vi "Execute Menu Item.vi"(7 "Device Ref in":T1 format="%.0x", 8 "error in (no error)":errorcluster, 9 "Coords":T2, 10 "ItemTag":string, 11 "CtlRef":refnum<vi>) -> (0 "error out":errorcluster)   [LabVIEW 2014, in "SLSC configuration System Explorer.lvlib"]
uses:
  SLSC configuration System Explorer.lvlib
  <vilib>/Utility/miscctls.llb/LVPoint32TypeDef.ctl
  <vilib>/NI Veristand/Custom Device API/Custom Device Item Ref.ctl
  Type Defs/Card Position.ctl
  Shared/SPI Utility/Slot #.ctl
  <vilib>/NI Veristand/Custom Device Tools/Custom Device Utility Library/NI VeriStand - Search for Item by Name.vi
  <vilib>/NI Veristand/Custom Device API/Custom Device API.lvlib
  <vilib>/NI Veristand/Custom Device Tools/Custom Device Utility Library/Custom Device Utility Library.lvlib
  Shared/SLSC configuration Shared.lvlib
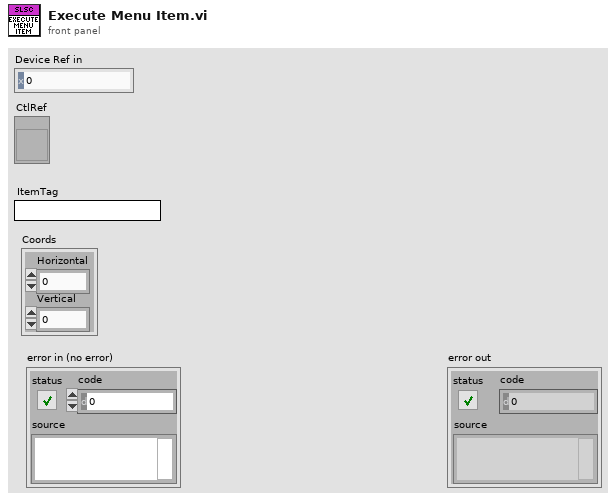
[diagram p1: front panel]
types:
  T1 = typedef "Custom Device API.lvlib/Custom Device Item Ref.ctl" = u64
  T2 = typedef "LVPoint32TypeDef.ctl" = cluster{"Horizontal":i32, "Vertical":i32}
  T3 = typedef "SLSC configuration Shared.lvlib/Card Position.ctl" = cluster{"Rack #":u8, "Slot #":T4}
  T4 = typedef "SLSC configuration Shared.lvlib/Slot #.ctl" = u8
  T5 = typedef "LVRowAndColumnTypeDef.ctl" = cluster{"Row":i32, "Column":i32}
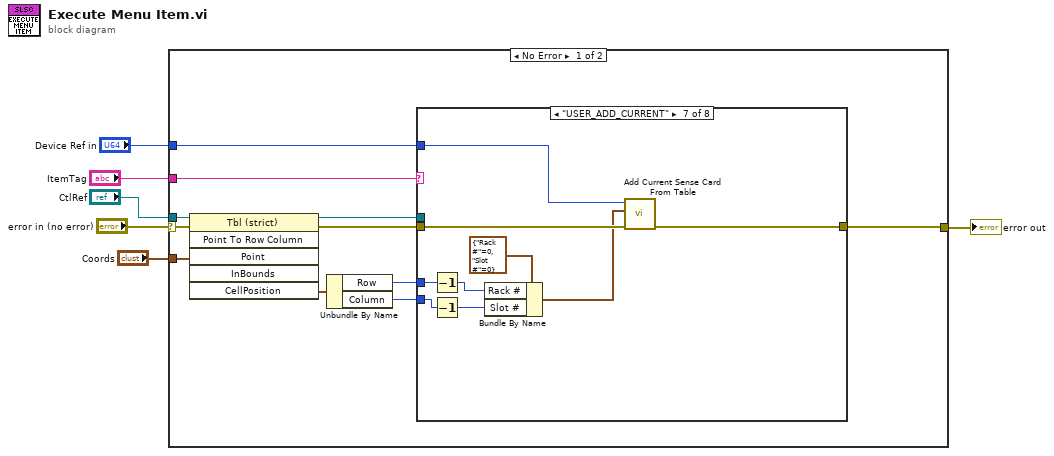
[diagram p0: block diagram]
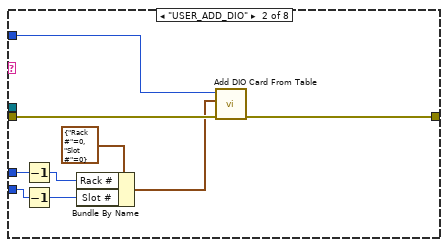
[diagram p3: hidden frame]
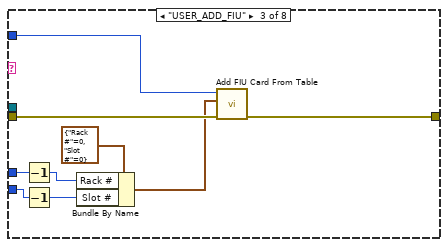
[diagram p4: hidden frame]
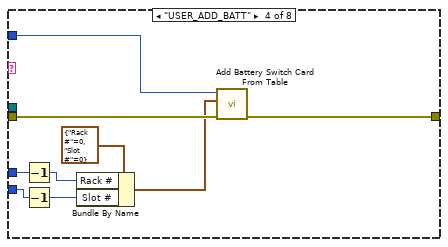
[diagram p5: hidden frame]
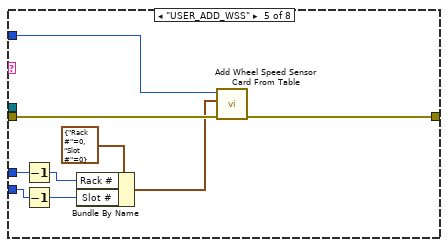
[diagram p6: hidden frame]
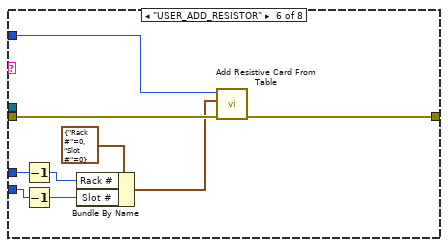
[diagram p7: hidden frame]
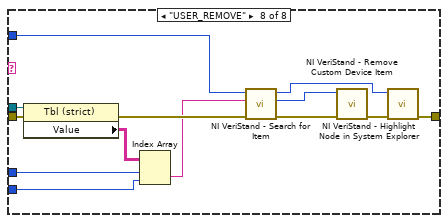
[diagram p8: hidden frame]
diagram:
  n1 = case shown="No Error" "error in (no error)" {
    selector: "error in (no error)" -> [w15 w86]
    tunnel: "ItemTag" -> [w17 _]
    tunnel: "CtlRef" -> [w16 _]
    tunnel: "Coords" -> [w14 _]
    tunnel: "Device Ref in" -> [w8 _]
    tunnel: [w7 w86] -> w1
    frame No Error {
      n2 = invoke class="Tbl (strict)" method="Point To Row Column"(reference=w16, error in=w15, "Point"=w14) -> (reference out=w13:refnum<vi>, error out=w12:errorcluster, "CellPosition"=w11:T5)  [unwired: 3 in, 3 out]
      n3 = Unbundle By Name(w11) -> ("Row"=w10:i32, "Column"=w9:i32)
      n4 = case shown="\"USER_ADD_CURRENT\"" w17 {
        tunnel: w13 -> [_ _ _ _ _ _ _ w85]
        tunnel: w12 -> [w18 w22 w31 w40 w49 w58 w67 w84]
        tunnel: w10 -> [_ w26 w35 w44 w53 w62 w71 w82]
        tunnel: w9 -> [_ w25 w34 w43 w52 w61 w70 w81]
        tunnel: w8 -> [_ w19 w29 w38 w47 w56 w65 w79]
        tunnel: [w18 w21 w30 w39 w48 w57 w66 w73] -> w7
        frame Default {
        }
        frame "USER_ADD_DIO" {
          n5 = Decrement(x=w26) -> (x-1=w24:i32)
          n6 = Decrement(x=w25) -> (x-1=w23:i32)
          n7 = Bundle By Name(cluster=T3 {"Rack #"=0, "Slot #"=0} ("Card Position"), "Rack #"=w24, "Slot #"=w23) -> (w20:T3)
          n8 = call "Add DIO Card From Table.vi"("error in (no error)"=w22, "Card Position"=w20, "Node Ptr"=w19) -> ("error out"=w21:errorcluster)  [unwired: 8 in]
        }
        frame "USER_ADD_FIU" {
          n9 = Decrement(x=w35) -> (x-1=w33:i32)
          n10 = Decrement(x=w34) -> (x-1=w32:i32)
          n11 = Bundle By Name(cluster=T3 {"Rack #"=0, "Slot #"=0} ("Card Position"), "Rack #"=w33, "Slot #"=w32) -> (w28:T3)
          n12 = call "Add FIU Card From Table.vi"("error in (no error)"=w31, "Card Position"=w28, "Node Ptr"=w29) -> ("error out"=w30:errorcluster)  [unwired: 8 in]
        }
        frame "USER_ADD_BATT" {
          n13 = Decrement(x=w44) -> (x-1=w42:i32)
          n14 = Decrement(x=w43) -> (x-1=w41:i32)
          n15 = Bundle By Name(cluster=T3 {"Rack #"=0, "Slot #"=0} ("Card Position"), "Rack #"=w42, "Slot #"=w41) -> (w37:T3)
          n16 = call "Add Battery Switch Card From Table.vi"("error in (no error)"=w40, "Card Position"=w37, "Node Ptr"=w38) -> ("error out"=w39:errorcluster)  [unwired: 8 in]
        }
        frame "USER_ADD_WSS" {
          n17 = Decrement(x=w53) -> (x-1=w51:i32)
          n18 = Decrement(x=w52) -> (x-1=w50:i32)
          n19 = Bundle By Name(cluster=T3 {"Rack #"=0, "Slot #"=0} ("Card Position"), "Rack #"=w51, "Slot #"=w50) -> (w46:T3)
          n20 = call "Add Wheel Speed Sensor Card From Table.vi"("error in (no error)"=w49, "Card Position"=w46, "Node Ptr"=w47) -> ("error out"=w48:errorcluster)  [unwired: 8 in]
        }
        frame "USER_ADD_RESISTOR" {
          n21 = Decrement(x=w62) -> (x-1=w60:i32)
          n22 = Decrement(x=w61) -> (x-1=w59:i32)
          n23 = Bundle By Name(cluster=T3 {"Rack #"=0, "Slot #"=0} ("Card Position"), "Rack #"=w60, "Slot #"=w59) -> (w55:T3)
          n24 = call "Add Resistive Card From Table.vi"("error in (no error)"=w58, "Card Position"=w55, "Node Ptr"=w56) -> ("error out"=w57:errorcluster)  [unwired: 8 in]
        }
        frame "USER_ADD_CURRENT" {
          n25 = Decrement(x=w71) -> (x-1=w69:i32)
          n26 = Decrement(x=w70) -> (x-1=w68:i32)
          n27 = Bundle By Name(cluster=T3 {"Rack #"=0, "Slot #"=0} ("Card Position"), "Rack #"=w69, "Slot #"=w68) -> (w64:T3)
          n28 = call "Add Current Sense Card From Table.vi"("error in (no error)"=w67, "Card Position"=w64, "Node Ptr"=w65) -> ("error out"=w66:errorcluster)  [unwired: 8 in]
        }
        frame "USER_REMOVE" {
          n29 = property class="Tbl (strict)"(reference=w85, error in=w84) -> (error out=w80:errorcluster, "Value"=w83:string[][])  [unwired: 1 out]
          n30 = Index Array(array=w83, index (row)=w82, index (col)=w81) -> (element=w78:string)
          n31 = call-poly <vilib>:"NI VeriStand - Search for Item.vi"("error in"=w80, "Item Name"=w78, "Section Ref in"=w79) -> ("error out"=w77:errorcluster, "Item Ref"=w76:T1, "Section Ref out"=w74:T1)  [unwired: 5 in, 1 out]
          n32 = call <vilib>:"NI VeriStand - Remove Custom Device Item.vi"("error in (no error)"=w77, "Item Ref in"=w76) -> ("error out"=w75:errorcluster)  [unwired: 8 in, 1 out]
          n33 = call <vilib>:"NI VeriStand - Highlight Node in System Explorer.vi"("error in (no error)"=w75, "Item Ref in"=w74) -> ("error out"=w73:errorcluster)  [unwired: 8 in, 1 out]
        }
      }
    }
    frame Error {
    }
  }
  "error out" <- w1
